vi "Update Memory.vi"(9 "value":refnum<class "Beam.lvclass">[](array[class]), 10 "Beam":refnum<class "Beam.lvclass">, 11 "Maze In":refnum<class "Maze.lvclass">) -> (3 "Maze Out":refnum<class "Maze.lvclass">)   [LabVIEW 2021, in "Maze.lvclass"]
uses:
  Maze.lvclass
  Beam/Beam.lvclass
  Maze.lvclass/Maze.ctl
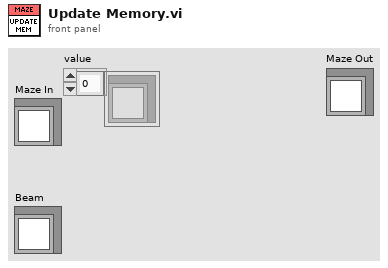
[diagram p1: front panel]
types:
  T1 = map{refnum<class "Beam.lvclass">, refnum<class "Beam.lvclass">[]}
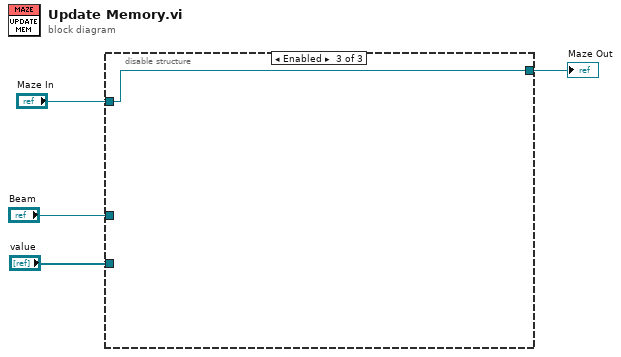
[diagram p0: block diagram]
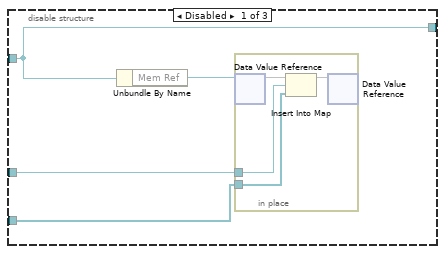
[diagram p2: hidden frame]
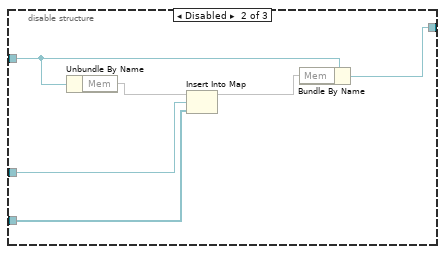
[diagram p3: hidden frame]
diagram:
  n1 = disable-structure shown="Enabled" {
    disable-tunnel: "Maze In" -> [w7 w18 w19]
    disable-tunnel: "Beam" -> [w6 w16 _]
    disable-tunnel: "value" -> [w5 w15 _]
    disable-tunnel: [w7 w13 w19] -> w1
    frame Disabled {
      n2 = Unbundle By Name(w7) -> ("Mem Ref"=w8:refnum<data-value>)
      n3 = in-place {
        in-place-border: w6 -> [w10]
        in-place-border: w5 -> [w9]
        n4 = in-place-dvr #1(w8) -> (w12:T1)  [unwired: 1 out]
        n5 = Insert Into Map(map in=w12, key=w10, value=w9) -> (map out=w11:T1)  [unwired: 2 out]
        n6 = in-place-dvr #1(w11) -> ()  [unwired: 2 out]
      }
    }
    frame Disabled {
      n7 = Unbundle By Name(w18) -> ("Mem"=w17:T1)
      n8 = Insert Into Map(map in=w17, key=w16, value=w15) -> (map out=w14:T1)  [unwired: 2 out]
      n9 = Bundle By Name(cluster=w18, "Mem"=w14) -> (w13:refnum<class "Maze.lvclass">)
    }
    frame Enabled {
    }
  }
  "Maze Out" <- w1
